vi "Create Pattern Script(ChipID).vi"(8 "error in (no error)":errorcluster, 10 "ChipID":u8, 11 "BML Pattern Creater in":refnum<class "BML Pattern Creater.lvclass">) -> (0 "error out":errorcluster, 2 "Script out":string, 3 "BML Pattern Creater out":refnum<class "BML Pattern Creater.lvclass">)   [LabVIEW 2018, in "BML Pattern Creater.lvlib" / "BML Pattern Creater.lvclass"]
uses:
  BML Pattern Creater.lvclass
  Interfaces/Protocol Interface.lvlibp/Interfaces/Protocol Interface/Pin State.ctl
  Interfaces/Protocol Interface.lvlibp/Interfaces/Protocol Interface/Protocol Interface.lvclass
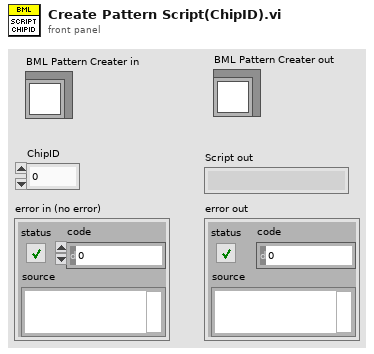
[diagram p1: front panel]
types:
  T1 = typedef "Protocol Interface.lvlibp/Protocol Interface.lvclass/Pin State.ctl" = enum16{"0", "1", "L", "H", "X", "V", "D", "M"}
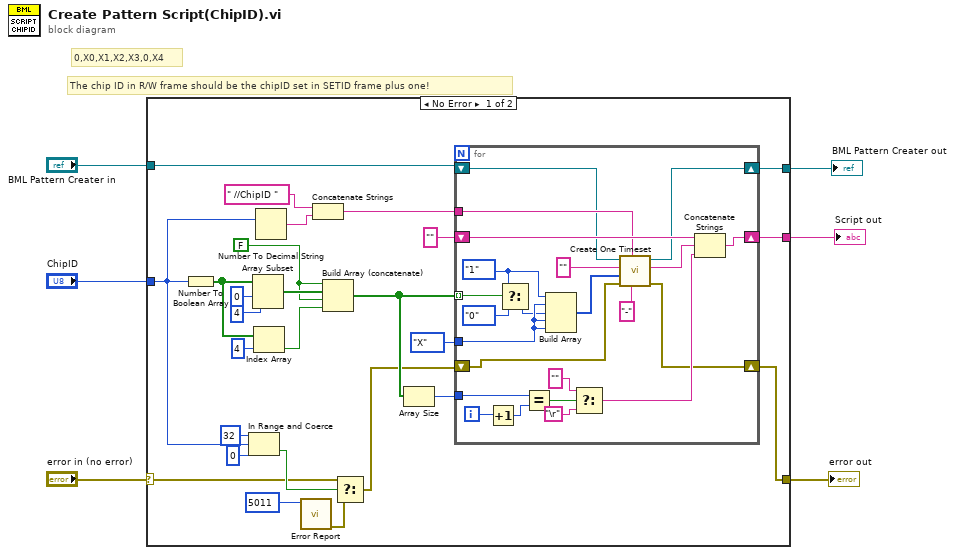
[diagram p0: block diagram]
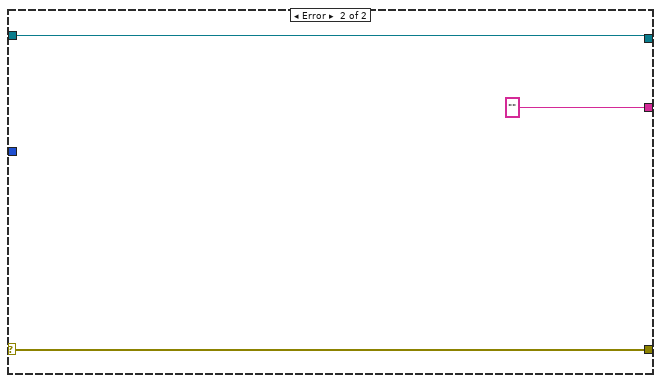
[diagram p2: hidden frame]
diagram:
  # "The chip ID in R/W frame should be the chipID set in SETID frame plus one!"
  # "0,X0,X1,X2,X3,0,X4"
  n1 = case shown="No Error" "error in (no error)" {
    selector: "error in (no error)" -> [w18 w57]
    tunnel: "ChipID" -> [w14 _]
    tunnel: [w24 ""] -> w4
    tunnel: [w7 w57] -> w3
    tunnel: "BML Pattern Creater in" -> [w10 w56]
    tunnel: [w9 w56] -> w1
    frame No Error {
      w26 = FALSE
      n2 = Number To Boolean Array(number=w14) -> (Boolean array=w30:bool[])
      n3 = In Range and Coerce(upper limit=u8 32, x=w14, lower limit=u8 0) -> (In Range?=w19:bool)  [unwired: 1 out]
      n4 = Array Subset(array=w30, index=0, length=4) -> (w28:bool[])
      n5 = Index Array(array=w30, index=4) -> (element=w27:bool)
      n6 = Number To Decimal String(number=w14) -> (decimal integer string=w16:string)  [unwired: 1 in]
      n7 = call "Error Report.vi"("Error Code"=i16 5011) -> ("error out"=w12:errorcluster)  [unwired: 10 in]
      n8 = Concatenate Strings(" //ChipID " ("Notes"), w16) -> (w15:string)
      n9 = Build Array (concatenate)(w26, w28, w26, w27) -> (w23:bool[])
      n10 = Select(t=w18, s=w19, f=w12) -> (s? t:f=w8:errorcluster)
      n11 = Array Size(array=w23) -> (size(s)=w22:i32)
      n12 = for {
        tunnel: w23 -> [w55] mode=indexing
        shift-right: [w54] -> w24
        shift-left: "" -> [w53]
        tunnel: w22 -> [w50]
        tunnel: Pin_State."X" ("PinState") -> [w45]
        tunnel: w15 -> [w41]
        shift-right: [w35] -> w9
        shift-left: w10 -> [w36]
        shift-right: [w33] -> w7
        shift-left: w8 -> [w34]
        i -> [w52]
        w43 = Pin_State."1" ("PinState")
        n13 = Increment(x=w52) -> (x+1=w51:i32)
        n14 = Select(t=w43, s=w55, f=Pin_State."0" ("PinState")) -> (s? t:f=w44:T1)
        n15 = Equal?(x=w50, y=w51) -> (x = y?=w49:bool)
        n16 = Build Array(w43, w45, w44, w45, w45) -> (w38:T1[])
        n17 = Select(t="", s=w49, f="\r") -> (s? t:f=w46:string)
        n18 = call-dynamic "Create One Timeset.vi"("timeset name"="-", "Notes"=w41, "error in (no error)"=w34, "Pin State"=w38, "opcode"="", "BML Pattern Creater in"=w36) -> ("error out"=w33:errorcluster, "string out"=w40:string, "BML Pattern Creater out"=w35:refnum<class "BML Pattern Creater.lvclass">)  [unwired: 3 in]
        n19 = Concatenate Strings(w53, w40, w46) -> (w54:string)
      }
    }
    frame Error {
    }
  }
  "Script out" <- w4
  "error out" <- w3
  "BML Pattern Creater out" <- w1
